vi "Tracepoint_DeleteCorruptStaleFile.vi"(8 "error in (no error)":errorcluster, 10 "file":path, 11 "Qbus in":refnum<class "Qbus.lvclass">) -> (0 "error out":errorcluster)   [LabVIEW 2017, in "FileManager.lvlib"]
uses:
  <vilib>/addons/InsightCM/Devices/Shared/Common/FileManager/FileManager.lvlib
  <vilib>/addons/Qbus/Qbus.lvclass
  <vilib>/addons/TraceLogger/TraceLogger.lvlib
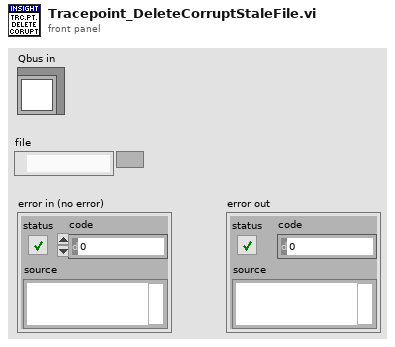
[diagram p1: front panel]
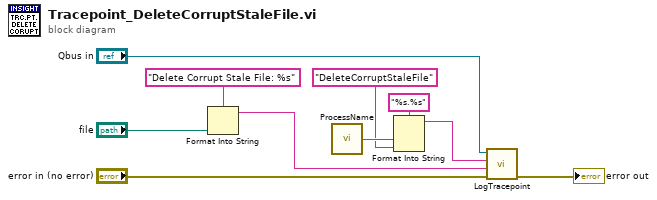
[diagram p0: block diagram]
diagram:
  n1 = Format Into String(format string="Delete Corrupt Stale File: %s", "file") -> (resulting string=w1:string)  [unwired: 2 in, 1 out]
  n2 = call <vilib>:"ProcessName.vi"() -> ("process name"=w7:string)  [unwired: 5 in]
  n3 = Format Into String(format string="%s.%s", w7, "DeleteCorruptStaleFile" ("tracepoint")) -> (resulting string=w4:string)  [unwired: 2 in, 1 out]
  n4 = call <vilib>:"LogTracepoint.vi"("error in (no error)"="error in (no error)", "log string"=w1, "tracepoint"=w4, "qbus in"="Qbus in") -> ("error out"=→"error out":errorcluster)  [unwired: 6 in, 1 out]
